vi "RegisteredMsgUpdate.vi"(8 "error in (no error)":errorcluster, 10 "Msgs":refnum<class "MailBoxMessage.lvclass">[](array[class]), 11 "MailboxManager in":refnum<class "MailboxManager.lvclass">) -> (0 "error out":errorcluster, 3 "MailboxManager out":refnum<class "MailboxManager.lvclass">)   [LabVIEW 2020, in "MailboxManager.lvlib" / "MailboxManager.lvclass"]
uses:
  MailboxManager.lvclass
  MailBoxMessage/MailBoxMessage.lvclass
  MailboxManager.lvclass/MailboxManager.ctl
  MailboxManager Messages/RegisteredMsgUpdate Msg/RegisteredMsgUpdate Msg.lvclass/RegisteredMsgUpdate Msg.ctl
  <vilib>/ActorFramework/Message Enqueuer/Message Enqueuer.lvclass/Message Enqueuer.ctl
  a186af84-16ea-4df5-a5b4-caa6cf910612.vi
  1c80b77f-6f19-468b-a1a1-57580433c264.vi
  <vilib>/ActorFramework/Message Enqueuer/Enqueue.vi
  MailboxManager Messages/RegisteredMsgUpdate Msg/RegisteredMsgUpdate Msg.lvclass
  C:/Program Files (x86)/National Instruments/LabVIEW 2020/vi.lib/ActorFramework/Message/Message.lvclass
  <vilib>/ActorFramework/Message Priority Queue/Priority Enqueue.vi
  <vilib>/ActorFramework/Message Enqueuer/Message Enqueuer.lvclass
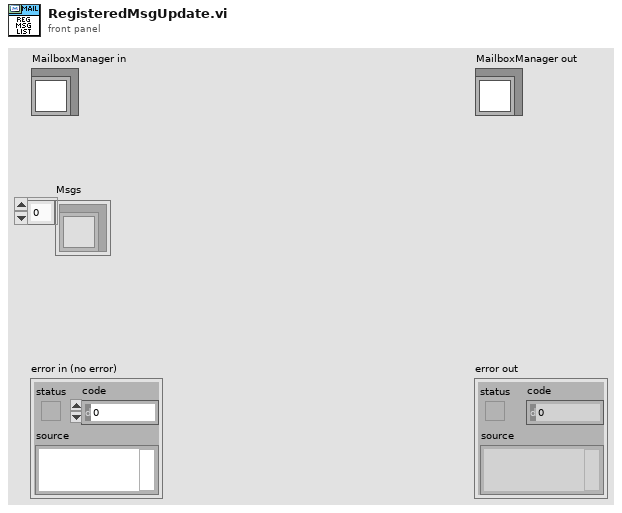
[diagram p1: front panel]
types:
  T1 = map{refnum<class "MailBoxMessage.lvclass">, refnum<class "Message Enqueuer.lvclass">[]}
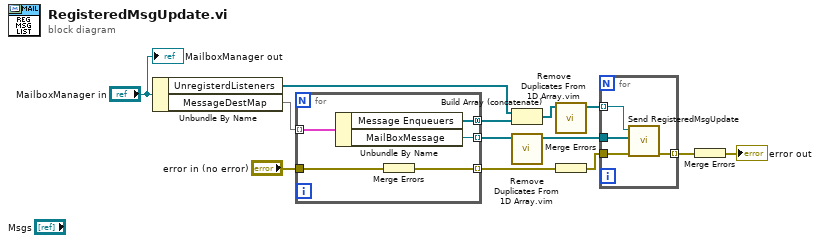
[diagram p0: block diagram]
diagram:
  n1 = Unbundle By Name("MailboxManager in") -> ("UnregisterdListeners"=w1:refnum<class "Message Enqueuer.lvclass">[], "MessageDestMap"=w12:T1)
  n2 = for {
    tunnel: w12 -> [w18] mode=indexing
    tunnel: "error in (no error)" -> [w15]
    tunnel: [w17] -> w10 mode=indexing
    tunnel: [w16] -> w9 mode=concatenating
    tunnel: [w14] -> w7 mode=indexing
    n3 = Unbundle By Name(w18) -> ("Message Enqueuers"=w16:refnum<class "Message Enqueuer.lvclass">[], "MailBoxMessage"=w14:refnum<class "MailBoxMessage.lvclass">)
    n4 = Merge Errors(w15) -> (w17:errorcluster)
  }
  n5 = Build Array (concatenate)(w1, w9) -> (w2:refnum<class "Message Enqueuer.lvclass">[])
  n6 = call "Remove Duplicates From 1D Array.vim"("array"=w7) -> ("array with duplicates removed"=w6:refnum<class "MailBoxMessage.lvclass">[])  [unwired: 10 in]
  n7 = call "Remove Duplicates From 1D Array.vim"("array"=w2) -> ("array with duplicates removed"=w8:refnum<class "Message Enqueuer.lvclass">[])  [unwired: 10 in]
  n8 = Merge Errors(w10) -> (w5:errorcluster)
  n9 = for {
    tunnel: w8 -> [w22] mode=indexing
    tunnel: w6 -> [w21]
    tunnel: w5 -> [w20]
    tunnel: [w19] -> w4 mode=indexing
    n10 = call "Send RegisteredMsgUpdate.vi"("error in (no error)"=w20, "Msgs"=w21, "Message Enqueuer"=w22) -> ("error out"=w19:errorcluster)  [unwired: 7 in, 1 out]
  }
  n11 = Merge Errors(w4) -> (→"error out":errorcluster)
  "MailboxManager out" <- "MailboxManager in"
